vi "Is Value within range.vi"(2 "%":dbl format="%#_g%", 5 "Target":dbl, 9 "Value":dbl) -> (6 "Greater?":bool, 8 "In Range?":bool, 10 "Lower?":bool)   [LabVIEW 2014]
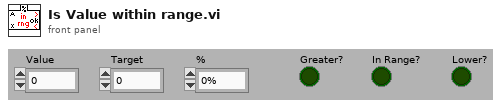
[diagram p1: front panel]
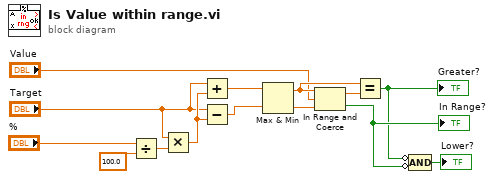
[diagram p0: block diagram]
diagram:
  n1 = Divide(x="%", y=100.0) -> (x/y=w4:dbl)
  n2 = Multiply(x="Target", y=w4) -> (x*y=w6:dbl)
  n3 = Add(x="Target", y=w6) -> (x+y=w7:dbl)
  n4 = Subtract(x="Target", y=w6) -> (x-y=w8:dbl)
  n5 = Max & Min(x=w7, y=w8) -> (max(x,y)=w11:dbl, min(x,y)=w3:dbl)
  n6 = In Range and Coerce(upper limit=w11, x="Value", lower limit=w3) -> (coerced(x)=w9:dbl, In Range?=w13:bool)
  "In Range?" <- w13
  n7 = Equal?(x=w11, y=w9) -> (x = y?=w12:bool)
  "Greater?" <- w12
  n8 = Compound Arithmetic op=AND(invert w12, invert w13) -> (→"Lower?":bool)
